vi "EQ_mono.vi"(1 "High 2400+ Hz (dB)":dbl(slide) scale=-10.0..10.0 scale format="%#_20g", 2 "Medium 200-2400 Hz (dB)":dbl(slide) scale=-10.0..10.0 scale format="%#_20g", 3 "Low 0-200 Hz (dB)":dbl(slide) scale=-10.0..10.0 scale format="%#_20g", 4 "Audio in":waveform(dbl)) -> (0 "output waveform":waveform(dbl))   [LabVIEW 2025]
uses:
  <vilib>/Analysis/3filter.llb/Filter Passband Type.ctl
  <vilib>/Analysis/3filter.llb/Butterworth Filter (DBL).vi
  <vilib>/Analysis/NI_AALBase.lvlib
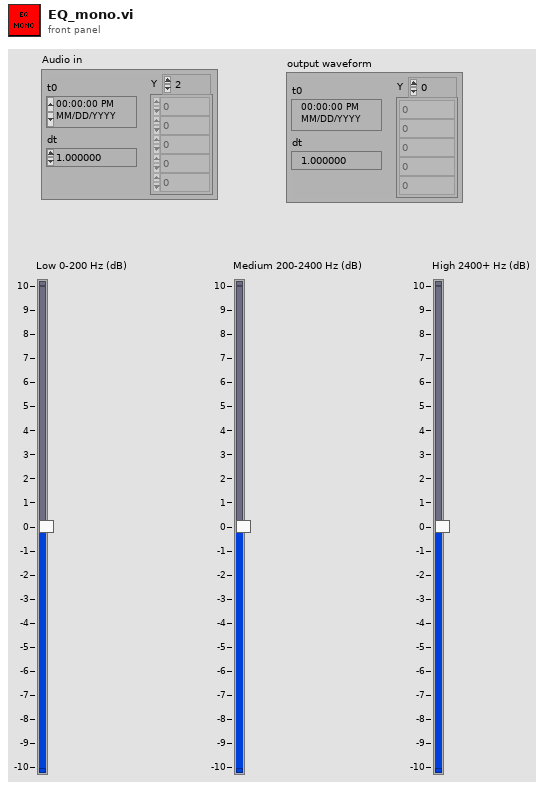
[diagram p1: front panel]
types:
  T1 = typedef "NI_AALBase.lvlib/Filter Passband Type.ctl" = enum32{"Lowpass", "Highpass", "Bandpass", "Bandstop"}
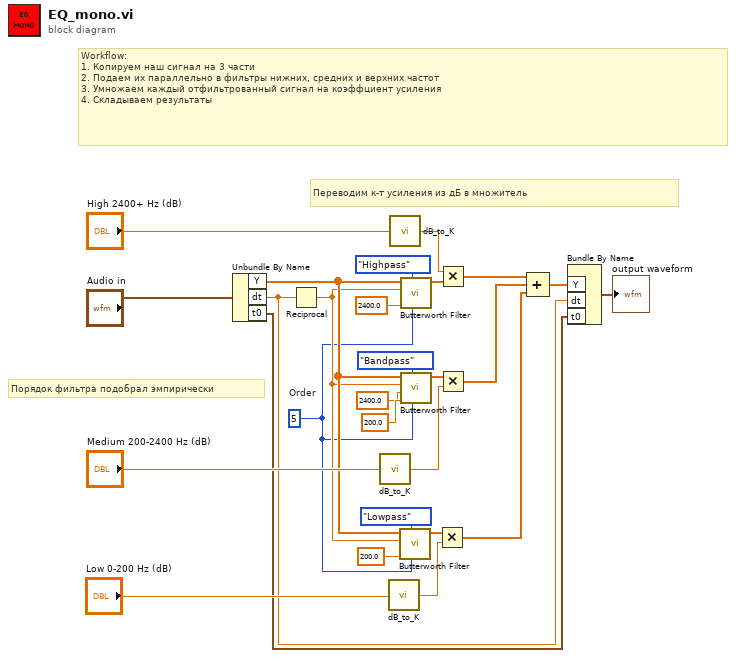
[diagram p0: block diagram]
diagram:
  w2 = i64 5  # Order
  # "Порядок фильтра подобрал эмпирически"
  # "Переводим к-т усиления из дБ в множитель"
  # "Workflow:\n1. Копируем наш сигнал на 3 части\n2. Подаем их параллельно в фильтры нижних, средних и верхних частот\n3. Умножаем каждый отфильтрованный сигнал на коэффциент усиления\n4. Складываем результаты"
  n1 = Unbundle By Name("Audio in") -> ("Y"=w8:dbl[], "dt"=w7:dbl, "t0"=w6:timestamp)
  n2 = Reciprocal(x=w7) -> (1/x=w3:dbl)
  n3 = call "dB_to_K.vi"("Усиление (дБ)"="Medium 200-2400 Hz (dB)") -> ("Коэффициент усиления"=w17:dbl)
  n4 = call "dB_to_K.vi"("Усиление (дБ)"="Low 0-200 Hz (dB)") -> ("Коэффициент усиления"=w16:dbl)
  n5 = call "dB_to_K.vi"("Усиление (дБ)"="High 2400+ Hz (dB)") -> ("Коэффициент усиления"=w18:dbl)
  n6 = call-poly <vilib>:"Butterworth Filter.vi"("order"=w2, "filter type"=Filter_Passband_Type."Lowpass", "low cutoff freq: fl"=200.0 ("high cutoff freq: fh"), "sampling freq: fs"=w3, "X"=w8) -> ("Filtered X"=w24:dbl[])  [unwired: 3 in, 1 out]
  n7 = call-poly <vilib>:"Butterworth Filter.vi"("order"=w2, "filter type"=Filter_Passband_Type."Highpass", "low cutoff freq: fl"=2400.0, "sampling freq: fs"=w3, "X"=w8) -> ("Filtered X"=w19:dbl[])  [unwired: 3 in, 1 out]
  n8 = call-poly <vilib>:"Butterworth Filter.vi"("order"=w2, "filter type"=Filter_Passband_Type."Bandpass", "low cutoff freq: fl"=200.0, "high cutoff freq: fh"=2400.0, "sampling freq: fs"=w3, "X"=w8) -> ("Filtered X"=w20:dbl[])  [unwired: 2 in, 1 out]
  n9 = Multiply(x=w24, y=w16) -> (x*y=w21:dbl[])
  n10 = Multiply(x=w18, y=w19) -> (x*y=w22:dbl[])
  n11 = Multiply(x=w20, y=w17) -> (x*y=w23:dbl[])
  n12 = Compound Arithmetic op=ADD(w22, w23, w21) -> (w5:dbl[])
  n13 = Bundle By Name("Y"=w5, "dt"=w7, "t0"=w6) -> (→"output waveform":waveform(dbl))  [unwired: 1 in]
